vi "Constructor_RQMHLogger.vi"(7 "RQMHLogger in":refnum<class "RQMHLogger.lvclass">, 8 "error in (no error)":errorcluster, 10 "Handles":refnum<class "HandleHolder.lvclass">[](array[class]), 11 "Name":string) -> (0 "error out":errorcluster, 3 "RQMHLogger out":refnum<class "RQMHLogger.lvclass">)   [LabVIEW 2024, in "RQMHLogger.lvclass"]
uses:
  RQMHLogger.lvclass
  RQMHLogger.lvclass/RQMHLogger.ctl
  HandleHolder/HandleHolder.lvclass
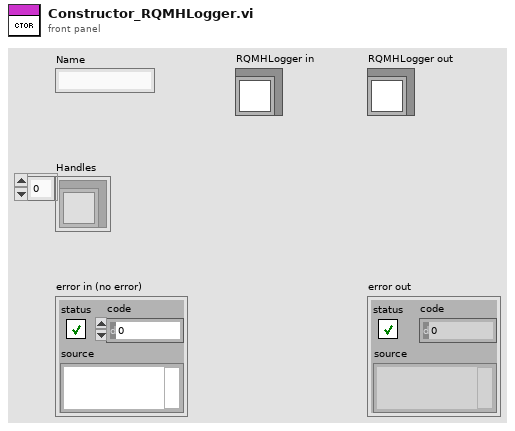
[diagram p1: front panel]
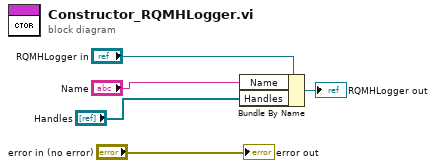
[diagram p0: block diagram]
diagram:
  n1 = Bundle By Name(cluster="RQMHLogger in", "Name"="Name", "Handles"="Handles") -> (→"RQMHLogger out":refnum<class "RQMHLogger.lvclass">)
  "error out" <- "error in (no error)"
